vi "Send Receive Notification.vi"(4 "Timeout":i32=-1, 6 "Write(T)":bool, 8 "error in (no error)":errorcluster, 10 "NotifierName":string, 11 "Data In":variant) -> (0 "error out":errorcluster, 2 "timed out?":bool, 3 "Data Out":variant)   [LabVIEW 2017]
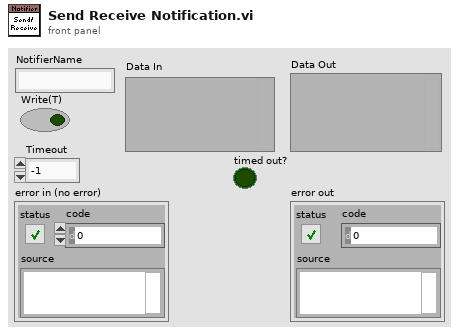
[diagram p1: front panel]
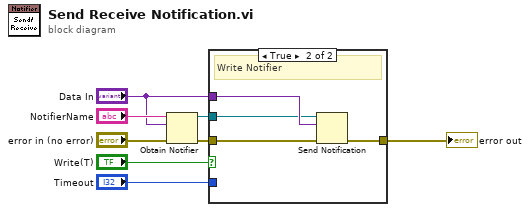
[diagram p0: block diagram]
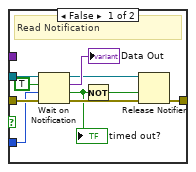
[diagram p2: hidden frame]
diagram:
  n1 = Obtain Notifier(name (unnamed)="NotifierName", notification data type="Data In", error in (no error)="error in (no error)") -> (notifier out=w7:refnum<notifier>, error out=w6:errorcluster)  [unwired: 1 in, 1 out]
  n2 = case shown="True" "Write(T)" {
    tunnel: w7 -> [w18 w20]
    tunnel: w6 -> [w17 w19]
    tunnel: [w12 w22] -> w1
    tunnel: "Data In" -> [_ w21]
    tunnel: "Timeout" -> [w15 _]
    frame False {
      # "Read Notification"
      n3 = Wait on Notification(notifier=w18, ignore previous (F)=TRUE, timeout in ms (-1)=w15, error in (no error)=w17) -> (notifier out=w14:refnum<notifier>, notification=→"Data Out":variant, timed out?=w11:bool, error out=w13:errorcluster)
      "timed out?" <- w11
      n4 = Not(x=w11) -> (.not. x?=w10:bool)
      n5 = Release Notifier(notifier=w14, force destroy? (F)=w10, error in (no error)=w13) -> (error out=w12:errorcluster)  [unwired: 2 out]
    }
    frame True {
      # "Write Notifier"
      n6 = Send Notification(notification=w21, notifier=w20, error in (no error)=w19) -> (error out=w22:errorcluster)  [unwired: 1 out]
    }
  }
  "error out" <- w1
